vi "alu_mux.vi"(1 "Control":T2, 2 "from_input":T1, 3 "from_acc":T1) -> (0 "Result":T3)   [LabVIEW 2013]
panel:
  # "R1"
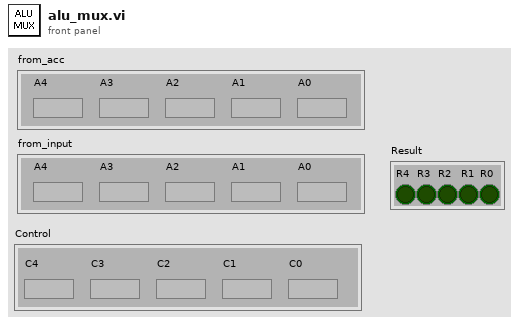
[diagram p1: front panel]
types:
  T1 = cluster{"A4":bool, "A3":bool, "A2":bool, "A1":bool, "A0":bool}
  T2 = cluster{"C4":bool, "C3":bool, "C2":bool, "C1":bool, "C0":bool}
  T3 = cluster{"R4":bool, "R3":bool, "R2":bool, bool, "R0":bool}
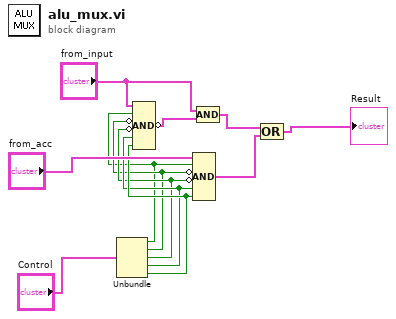
[diagram p0: block diagram]
diagram:
  n1 = Unbundle("Control") -> ("C4"=w1:bool, "C3"=w2:bool, "C2"=w3:bool, "C1"=w4:bool, "C0"=w5:bool)
  n2 = Compound Arithmetic op=AND("from_input", w1, invert w2, invert w3, w4, w5) -> (invert w8:T1)
  n3 = Compound Arithmetic op=AND("from_acc", w1, invert w2, invert w3, w4, w5) -> (w10:T1)
  n4 = Compound Arithmetic op=AND("from_input", w8) -> (w7:T1)
  n5 = Compound Arithmetic op=OR(w7, w10) -> (→"Result":T1)
